vi "oax_AI Configuration Error Handling.vi"(8 "error in":errorcluster, 11 "task in":refnum<k21>) -> (0 "error out":errorcluster, 3 "task out":refnum<k21>)   [LabVIEW 2017]
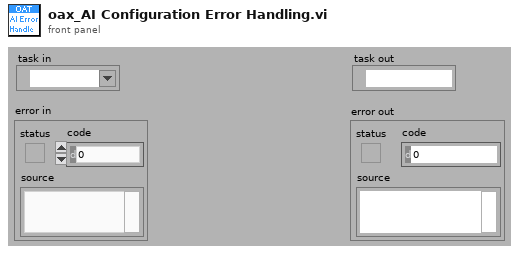
[diagram p1: front panel]
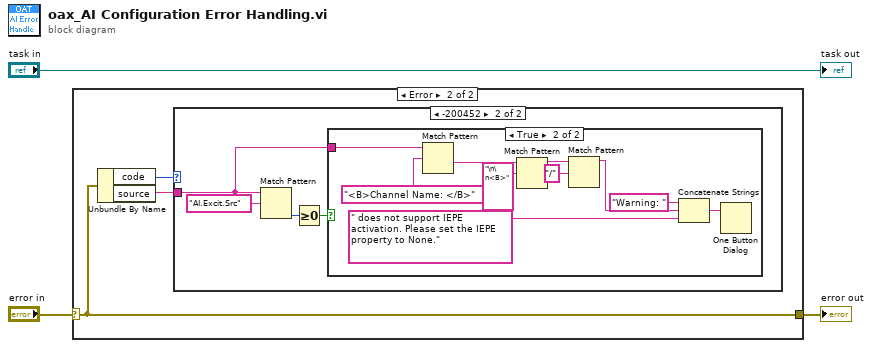
[diagram p0: block diagram]
diagram:
  n1 = case shown="Error" "error in" {
    selector: "error in" -> [w4 w7]
    tunnel: [w4 w7] -> w3
    frame No Error {
    }
    frame Error {
      n2 = Unbundle By Name(w7) -> ("code"=w6:i32, "source"=w5:string)
      n3 = case shown="-200452" w6 {
        tunnel: w5 -> [_ w8]
        frame 0, Default {
        }
        frame -200452 {
          n4 = Match Pattern(string=w8, regular expression="AI.Excit.Src") -> (offset past match=w10:i32)  [unwired: 1 in, 3 out]
          n5 = Greater Or Equal To 0?(x=w10) -> (x >= 0?=w9:bool)
          n6 = case shown="True" w9 {
            tunnel: w8 -> [_ w15]
            frame False {
            }
            frame True {
              n7 = Match Pattern(string=w15, regular expression="<B>Channel Name: </B>") -> (after substring=w20:string)  [unwired: 1 in, 3 out]
              n8 = Match Pattern(string=w20, regular expression="\n\n<B>") -> (before substring=w14:string)  [unwired: 1 in, 3 out]
              n9 = Match Pattern(string=w14, regular expression="/") -> (before substring=w12:string)  [unwired: 1 in, 3 out]
              n10 = Concatenate Strings("Warning: " ("regular expression"), w12, " does not support IEPE activation. Please set the IEPE property to None." ("string")) -> (w17:string)
              n11 = One Button Dialog(message=w17) -> ()  [unwired: 1 in, 1 out]
            }
          }
        }
      }
    }
  }
  "error out" <- w3
  "task out" <- "task in"
